vi "MaxPIDMain.vi"(6 "Reset":bool, 7 "Output Range":cluster{"Max Output":dbl, "Min Output":dbl} {"Min Output" format="%.2f"; "Max Output" format="%.2f"}, 8 "dt (s)":dbl=-1.0 format="%.3f", 9 "PID gains":T1={"proportional gain (Kc)"=1.0, "integral gain (Ki)"=0.01, "derivative gain (Kd)"=0.0} {"derivative gain (Kd)" format="%.3f"; "integral gain (Ki)" format="%.3f"; "proportional gain (Kc)" format="%.3f"}, 10 "process variable":dbl format="%.2f", 11 "setpoint":dbl format="%.2f") -> (0 "dt out (s)":dbl format="%.3f", 3 "Output":dbl format="%.3f")   [LabVIEW 2012]
panel:
  out "D action":dbl
  out "I action":dbl
  out "P action":dbl
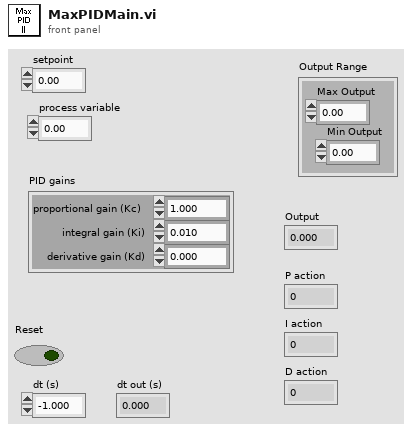
[diagram p1: front panel]
types:
  T1 = cluster{"proportional gain (Kc)":dbl, "integral gain (Ki)":dbl, "derivative gain (Kd)":dbl}
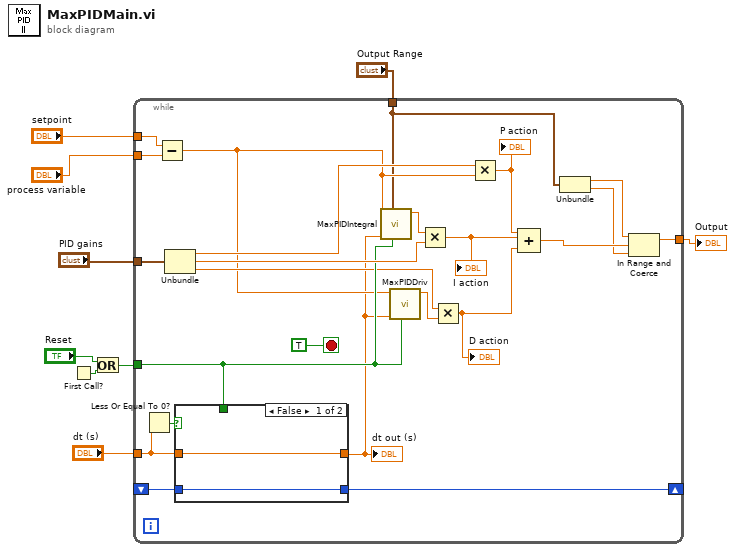
[diagram p0: block diagram]
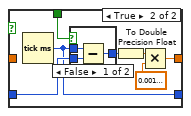
[diagram p2: hidden frame]
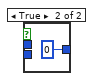
[diagram p3: hidden frame]
diagram:
  n1 = First Call?() -> (First Call?: T/F=w6:bool)
  n2 = Or(x="Reset", y=w6) -> (x .or. y?=w4:bool)
  n3 = while {
    tunnel: "dt (s)" -> [w31]
    tunnel: w4 -> [w22]
    shift-right: [w29] -> _
    shift-left: _ -> [w30]
    tunnel: "setpoint" -> [w28]
    tunnel: "process variable" -> [w27]
    tunnel: "PID gains" -> [w26]
    tunnel: "Output Range" -> [w15]
    tunnel: [w11] -> w1
    stop <- TRUE stop-if-true
    n4 = Less Or Equal To 0?(x=w31) -> (x <= 0?=w32:bool)
    n5 = Subtract(x=w28, y=w27) -> (x-y=w19:dbl)
    n6 = Unbundle(w26) -> ("proportional gain (Kc)"=w25:dbl, "integral gain (Ki)"=w23:dbl, "derivative gain (Kd)"=w20:dbl)
    n7 = case shown="False" w32 {
      tunnel: [w35 w39] -> w18
      tunnel: w30 -> [w34 w38]
      tunnel: [w34 w37] -> w29
      tunnel: w31 -> [w35 _]
      tunnel: w22 -> [_ w36]
      frame False {
      }
      frame True {
        n8 = Tick Count (ms)() -> (millisecond timer value=w37:u32)
        n9 = case shown="False" w36 {
          tunnel: [w45 u32 0] -> w41
          tunnel: w38 -> [w44 _]
          tunnel: w37 -> [w43 _]
          frame False {
            n10 = Subtract(x=w43, y=w44) -> (x-y=w45:u32)
          }
          frame True {
          }
        }
        n11 = To Double Precision Float(number=w41) -> (double precision float=w40:dbl)
        n12 = Multiply(x=w40, y=0.0010000000474974513) -> (x*y=w39:dbl)
      }
    }
    "dt out (s)" <- w18
    n13 = call "MaxPIDIntegral.vi"("Reset"=w22, "Output Range"=w15, "dt (s)"=w18, "Error"=w19) -> ("Integral"=w24:dbl)  [unwired: 7 in]
    n14 = call "MaxPIDDriv.vi"("Reset"=w22, "dt (s)"=w18, "Error"=w19) -> ("Drivative"=w21:dbl)  [unwired: 8 in]
    n15 = Multiply(x=w24, y=w23) -> (x*y=w16:dbl)
    "I action" <- w16
    n16 = Multiply(x=w20, y=w21) -> (x*y=w10:dbl)
    "D action" <- w10
    n17 = Multiply(x=w25, y=w19) -> (x*y=w17:dbl)
    "P action" <- w17
    n18 = Compound Arithmetic op=ADD(w17, w16, w10) -> (w13:dbl)
    n19 = Unbundle(w15) -> ("Max Output"=w14:dbl, "Min Output"=w12:dbl)
    n20 = In Range and Coerce(upper limit=w14, x=w13, lower limit=w12) -> (coerced(x)=w11:dbl)  [unwired: 1 out]
  }
  "Output" <- w1
